vi "Create Server Key.vi"(8 "error in (no error)":errorcluster, 11 "Server Fixture in":refnum<class "Server Fixture.lvclass">) -> (0 "error out":errorcluster, 3 "Server Fixture out":refnum<class "Server Fixture.lvclass">)   [LabVIEW 2013, in "libssh2_integration_tests.lvlib" / "Server Fixture.lvclass"]
uses:
  Server Fixture.lvclass
  Server Fixture.lvclass/Server Fixture.ctl
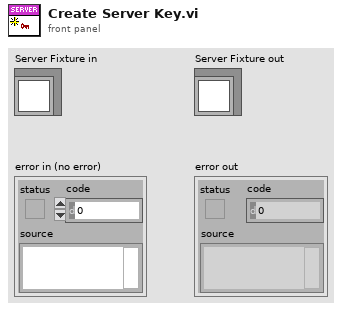
[diagram p1: front panel]
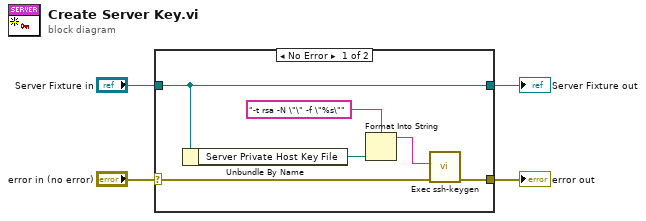
[diagram p0: block diagram]
diagram:
  n1 = case shown="No Error" "error in (no error)" {
    selector: "error in (no error)" -> [w6 w12]
    tunnel: [w5 w12] -> w3
    tunnel: [w7 w11] -> w1
    tunnel: "Server Fixture in" -> [w7 w11]
    frame No Error {
      n2 = Unbundle By Name(w7) -> ("Server Private Host Key File"=w8:path)
      n3 = Format Into String(format string="-t rsa -N \"\" -f \"%s\"", w8) -> (resulting string=w9:string)  [unwired: 2 in, 1 out]
      n4 = call "Exec ssh-keygen.vi"("error in (no error)"=w6, "arguments"=w9) -> ("error out"=w5:errorcluster)  [unwired: 9 in]
    }
    frame Error {
    }
  }
  "error out" <- w3
  "Server Fixture out" <- w1
